vi "Samplepoint Anzahl.vi"(6 "Aktion":enum16{"lesen", "Ref schreiben", "SP setzen"}(ring), 7 "PNS aktiv":bool, 8 "error in (no error)":errorcluster caption="Fehler (Eingang, kein Fehler)", 9 "Samplepoint Referenz":refnum<vi>) -> (0 "error out":errorcluster caption="Fehler (Ausgang)", 1 "Anzahl SP":i32)   [LabVIEW 2020, in "allgemeine Sub-VIs.lvlib"]
doc: "Setzt das Auswahlfeld für SP über die ControlRefernz im Haupt VI.\nVon FUM übernommen und mit #DynPNS erweitert.\nAktion:\ninit ... setzen der Referenz des Auswahlfeldes aus dem HauptVI\nSP setzen ... PNS aktiv mit geben, Gerätekenung wird ausgewertet und Anzahl der SP ermittelt, Auswahlfeld Ring Texte gesetzt. Hier ist auch der einzige zentrale Punkt, wo die Anzahl der SPs der Versa selbst gesetzt wird, wenn PNS inaktiv.\nSetzt den bereits ausgewählten Wert auf den maximalen, falls höher - signalisierend.\nlesen ... Anzahl SP - zum Begrenzen für maximale SP Auswahl in Funktionstasten setzen (z.B. via AK)\n\nRIW - 24.08.2018"
uses:
  allgemeine Sub-VIs.lvlib
  PNS/Aktionen FGV Loopkennung.ctl
  PNS/PNS.lvlib
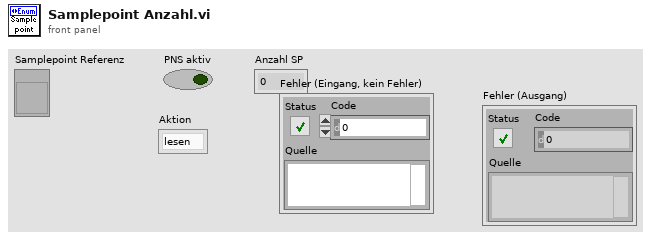
[diagram p1: front panel]
types:
  T1 = typedef "PNS.lvlib/Aktionen FGV Loopkennung.ctl" = enum16{"lesen", "schreiben"}
  T2 = typedef "PNS.lvlib/PNS Geraetekennung.ctl" = cluster{"Loops":string[], "Gerätetype":string, "Loopkennung":u16[], "Seriennummer":string, "Geraetekennung":u16, "SoftWare Version":string, "LP Kennung":u16}
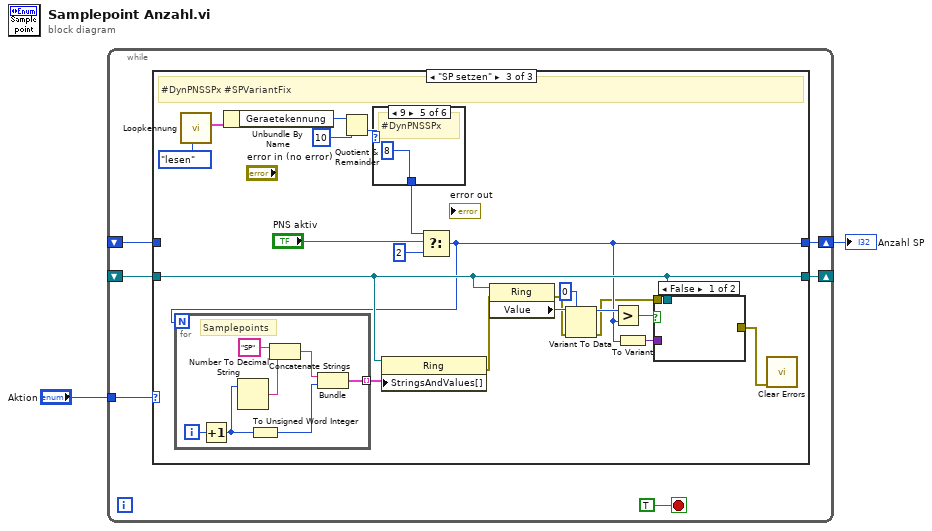
[diagram p0: block diagram]
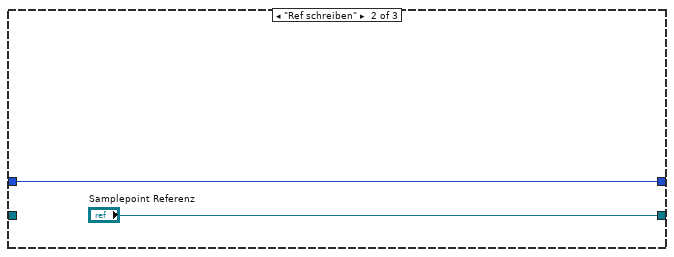
[diagram p3: hidden frame]
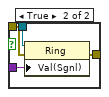
[diagram p4: hidden frame]
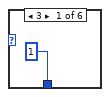
[diagram p5: hidden frame]
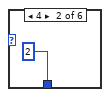
[diagram p6: hidden frame]
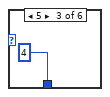
[diagram p7: hidden frame]
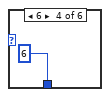
[diagram p8: hidden frame]
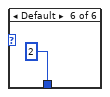
[diagram p9: hidden frame]
diagram:
  n1 = while {
    tunnel: "Aktion" -> [w7]
    shift-right: [w6] -> _
    shift-left: _ -> [w5]
    shift-right: [w4] -> w1
    shift-left: _ -> [w3]
    stop <- TRUE stop-if-true
    n2 = case shown="\"SP setzen\"" w7 {
      tunnel: [w10 "Samplepoint Referenz" w19] -> w6
      tunnel: w5 -> [w10 _ w19]
      tunnel: [w9 w11 w16] -> w4
      tunnel: w3 -> [w9 w11 _]
      frame "lesen", Default {
      }
      frame "Ref schreiben" {
      }
      frame "SP setzen" {
        # "#DynPNSSPx #SPVariantFix"
        n3 = call "Loopkennung.vi"("Aktion"=Aktionen_FGV_Loopkennung."lesen") -> ("LoopGeraetekennung"=w29:T2)  [unwired: 9 in, 1 out]
        n4 = Unbundle By Name(w29) -> ("Geraetekennung"=w28:u16)
        n5 = Quotient & Remainder(x=w28, y=u16 10) -> (floor(x/y)=w26:u16)  [unwired: 1 out]
        n6 = case shown="9" w26 {
          tunnel: [1 ("t") 2 ("t") 4 ("t") 6 ("t") 8 ("t") 2 ("t")] -> w24
          frame 3 {
          }
          frame 4 {
          }
          frame 5 {
          }
          frame 6 {
          }
          frame 9 {
            # "#DynPNSSPx"
          }
          frame Default {
          }
        }
        n7 = Select(t=w24, s="PNS aktiv", f=2) -> (s? t:f=w16:i32)
        n8 = for {
          N: w16 -> [_]
          tunnel: [w44] -> w32 mode=indexing
          i -> [w49]
          # "Samplepoints"
          n9 = Increment(x=w49) -> (x+1=w43:i32)
          n10 = Number To Decimal String(number=w43) -> (decimal integer string=w47:string)  [unwired: 1 in]
          n11 = To Unsigned Word Integer(number=w43) -> (unsigned 16bit integer=w45:u16)
          n12 = Concatenate Strings("SP", w47) -> (w46:string)
          n13 = Bundle(w46, w45) -> (w44:cluster{string, u16})  [unwired: 1 in]
        }
        n14 = property class="Ring"(reference=w19, "StringsAndValues[]"=w32) -> (error out=w18:errorcluster)  [unwired: 1 in, 1 out]
        n15 = property class="Ring"(reference=w19, error in=w18) -> (error out=w14:errorcluster, "Value"=w23:variant)  [unwired: 1 out]
        n16 = Variant To Data(error in=w14, type=0 ("f"), Variant=w23) -> (data=w21:i32, error out=w13:errorcluster)
        n17 = Greater?(x=w21, y=w16) -> (0:w20:bool)
        n18 = To Variant(anything=w16) -> (Variant=w17:variant)
        n19 = case shown="False" w20 {
          tunnel: w19 -> [_ w36]
          tunnel: w17 -> [_ w35]
          tunnel: w13 -> [_ w34]
          tunnel: [_ w33] -> w15
          frame False {
          }
          frame True {
            n20 = property class="Ring"(reference=w36, error in=w34, "Val(Sgnl)"=w35) -> (error out=w33:errorcluster)  [unwired: 1 out]
          }
        }
        n21 = call <vilib>:"Clear Errors.vi"("error in (no error)"=w15) -> ()  [unwired: 5 in, 2 out]
      }
    }
  }
  "Anzahl SP" <- w1
